vi "Periodic Tasks.vi"(8 "error in":errorcluster) -> ()   [LabVIEW 2015]
doc: "This VI runs in parallel to other tasks. It can contain as many user-defined periodic loops as you need. These can carry out PID or other sorts of timed response."
uses:
  <vilib>/Rock Robotics/WPI/Utilities/WPI_GetSetVariantRefNum.vi
  Mr. Thayer.vi
  Mr. Thayer 2.0.vi
  <vilib>/Rock Robotics/WPI/RobotDrive/WPI_RobotDriveArcadeDrive_Standard(NoSaturation).vi
  Global 3.vi
  Global 4.vi
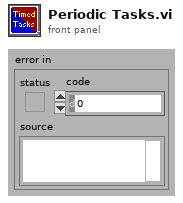
[diagram p1: front panel]
types:
  T1 = typedef "WPI_ServoDeviceRef.ctl" = cluster{"DeviceStatus":errorcluster, "PWM Channel":T2, "DeadBand":T3}
  T2 = typedef "FPGA_DIOPWMChannel.ctl" = enum8{"PWM 0", "PWM 1", "PWM 2", "PWM 3", "PWM 4", "PWM 5", "PWM 6", "PWM 7", "PWM 8", "PWM 9", "PWM MXP 0", "PWM MXP 1", "PWM MXP 2", "PWM MXP 3", "PWM MXP 4", "PWM MXP 5", "PWM MXP 6", "PWM MXP 7", "PWM MXP 8", "PWM MXP 9", "Invalid"}
  T3 = typedef "WPI_PWMDeadband.ctl" = cluster{"Name":string, "maxPositivePwm":i32, "minPositivePwm":i32, "centerPwm":i32, "maxNegativePwm":i32, "minNegativePwm":i32, "angularRange":u16}
  T4 = typedef "WPI_JoystickDevRef.ctl" = cluster{"Device":T5}
  T5 = typedef "WPI_JoystickDeviceEnum.ctl" = enum16{"USB 0", "USB 1", "USB 2", "USB 3", "USB 4", "USB 5"}
  T6 = typedef "WPI_RobotDriveDevRef.ctl" = cluster{"DevStatus":errorcluster, "Motors[]":T7[], "Square Inputs":bool, "Max Output":dbl}
  T7 = typedef "WPI_MotorControlDeviceRef.ctl" = cluster{"DeviceStatus":errorcluster, "Type":T8, "PWM":cluster{"PWM Channel":T2, "DeadBand":T3}, "CAN":cluster{"Device Number":u8, "Control Mode":T9, "Semaphore":T10, "Max Vout":dbl, "TalonSRX Control Mode":T11}, "Invert":bool}
  T8 = typedef "WPI_MotorControlType.ctl" = enum16{"PWM", "CAN", "CANTalonSRX"}
  T9 = typedef "WPI_CANJaguar_ControlMode.ctl" = enum8{"Percent VBus", "Current", "Speed", "Position", "Voltage"}
  T10 = typedef "Semaphore RefNum" = refnum<k1>
  T11 = typedef "WPI_CANTalonSRX_APIControlMode.ctl" = enum8{"Percent VBus", "Speed", "Position", "Slave", "Unchanged / Invalid", "Voltage Compensation", "Current", "Motion Profile"}
  T12 = cluster{"JoystickDevRef":T4, "RobotDriveDevRef":T6}
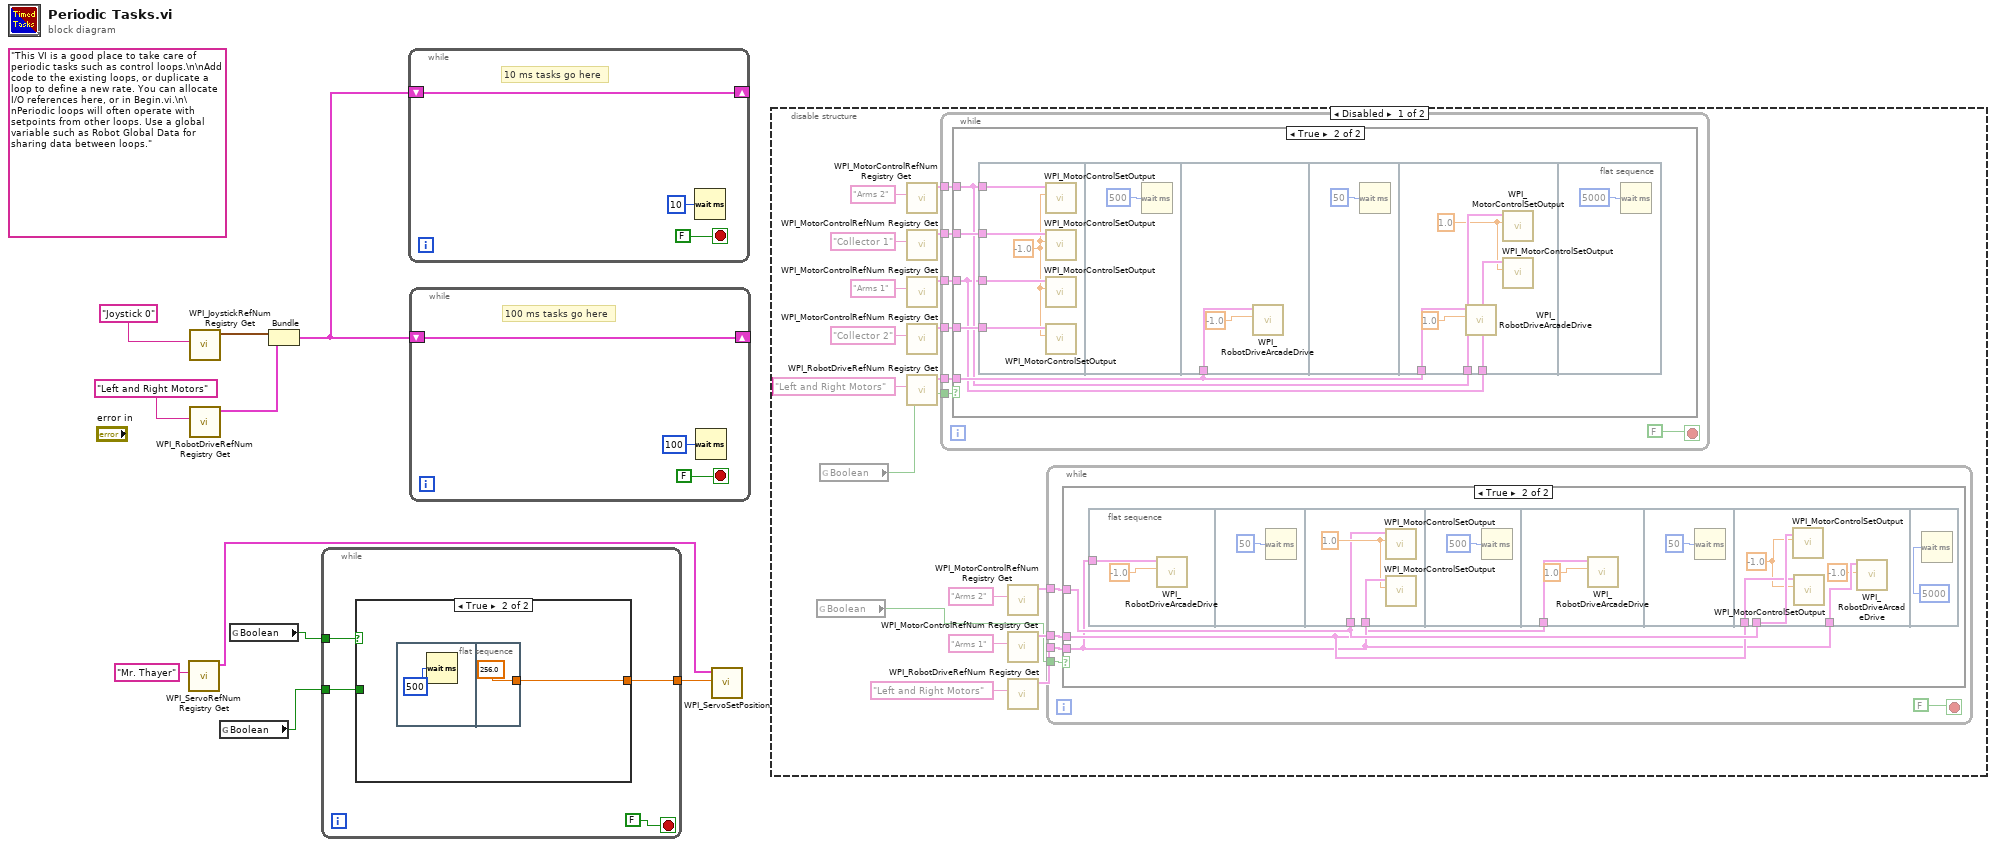
[diagram p0: block diagram]
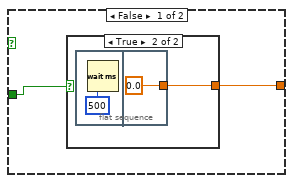
[diagram p2: hidden frame]
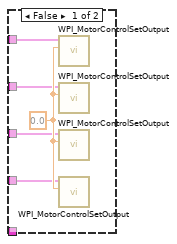
[diagram p4: hidden frame]
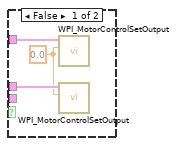
[diagram p5: hidden frame]
diagram:
  (unwired) "This VI is a good place to take care of periodic tasks such as control loops.\n\nAdd code to the existing loops, or duplicate a loop to define a new rate. You can allocate I/O references here, or in Begin.vi.\n\nPeriodic loops will often operate with setpoints from other loops. Use a global variable such as Robot Global Data for sharing data between loops."
  n1 = call <vilib>:"WPI_ServoRefNum Registry Get.vi"("refnum name"="Mr. Thayer") -> ("ServoDeviceRef"=w1:T1)  [unwired: 9 in, 1 out]
  n2 = call <vilib>:"WPI_JoystickRefNum Registry Get.vi"("refnum name"="Joystick 0") -> ("JoystickDevRef"=w8:T4)  [unwired: 1 in, 9 out]
  n3 = call <vilib>:"WPI_RobotDriveRefNum Registry Get.vi"("refnum name"="Left and Right Motors") -> ("RobotDriveDevRef"=w7:T6)  [unwired: 1 in, 9 out]
  n4 = global read "Mr. Thayer 2.0.vi" "Boolean"() -> (w3:bool)
  n5 = global read "Mr. Thayer.vi" "Boolean"() -> (w5:bool)
  n6 = Bundle("JoystickDevRef"=w8, "RobotDriveDevRef"=w7) -> (w6:T12)  [unwired: 1 out]
  n7 = while {
    tunnel: w5 -> [w14]
    tunnel: w3 -> [w13]
    tunnel: [w12] -> w2
    stop <- FALSE stop-if-true
    n8 = case shown="True" w14 {
      tunnel: w13 -> [w16 _]
      tunnel: [w15 w20] -> w12
      frame False {
        n9 = case shown="True" w16 {
          tunnel: [_ w17] -> w15
          frame False {
          }
          frame True {
            n10 = flat-sequence {
              tunnel: [0.0] -> w17
              frame #0 {
                n11 = Wait (ms)(milliseconds to wait=500) -> ()  [unwired: 1 out]
              }
              frame #1 {
              }
            }
          }
        }
      }
      frame True {
        n12 = flat-sequence {
          tunnel: [256.0] -> w20
          frame #0 {
            n13 = Wait (ms)(milliseconds to wait=500) -> ()  [unwired: 1 out]
          }
          frame #1 {
          }
        }
      }
    }
  }
  n14 = while {
    shift-right: [w23] -> _
    shift-left: w6 -> [w23]
    stop <- FALSE stop-if-true
    # "10 ms tasks go here"
    n15 = Wait (ms)(milliseconds to wait=u32 10) -> ()  [unwired: 1 out]
  }
  n16 = while {
    shift-right: [w26] -> _
    shift-left: w6 -> [w26]
    stop <- FALSE stop-if-true
    # "100 ms tasks go here"
    n17 = Wait (ms)(milliseconds to wait=u32 100) -> ()  [unwired: 1 out]
  }
  n18 = call <vilib>:"WPI_ServoSetPosition.vi"("Position"=w2, "ServoDeviceRef"=w1) -> ()  [unwired: 8 in, 2 out]
  n19 = disable-structure shown="Disabled" {
    frame Disabled {
      n20 = global read "Global 4.vi" "Boolean"() -> (w29:bool)
      n21 = global read "Global 3.vi" "Boolean"() -> (w36:bool)
      n22 = call <vilib>:"WPI_MotorControlRefNum Registry Get.vi"("refnum name"="Arms 2") -> ("MotorControlDevRef"=w43:T7)  [unwired: 9 in, 1 out]
      n23 = call <vilib>:"WPI_MotorControlRefNum Registry Get.vi"("refnum name"="Collector 1") -> ("MotorControlDevRef"=w46:T7)  [unwired: 9 in, 1 out]
      n24 = call <vilib>:"WPI_MotorControlRefNum Registry Get.vi"("refnum name"="Arms 1") -> ("MotorControlDevRef"=w44:T7)  [unwired: 9 in, 1 out]
      n25 = call <vilib>:"WPI_MotorControlRefNum Registry Get.vi"("refnum name"="Collector 2") -> ("MotorControlDevRef"=w45:T7)  [unwired: 9 in, 1 out]
      n26 = call <vilib>:"WPI_RobotDriveRefNum Registry Get.vi"("refnum name"="Left and Right Motors") -> ("RobotDriveDevRef"=w37:T6)  [unwired: 9 in, 1 out]
      n27 = while {
        tunnel: w46 -> [w53]
        tunnel: w45 -> [w52]
        tunnel: w44 -> [w51]
        tunnel: w43 -> [w50]
        tunnel: w37 -> [w49]
        tunnel: w36 -> [w48]
        stop <- FALSE stop-if-true
        n28 = case shown="True" w48 {
          tunnel: w53 -> [w57 w63]
          tunnel: w52 -> [w56 w62]
          tunnel: w51 -> [w55 w59]
          tunnel: w50 -> [w54 w60]
          tunnel: w49 -> [_ w61]
          frame False {
            w58 = 0.0
            n29 = call <vilib>:"WPI_MotorControlSetOutput.vi"("Output"=w58, "MotorControlDevRef"=w54) -> ()  [unwired: 7 in, 3 out]
            n30 = call <vilib>:"WPI_MotorControlSetOutput.vi"("Output"=w58, "MotorControlDevRef"=w57) -> ()  [unwired: 7 in, 3 out]
            n31 = call <vilib>:"WPI_MotorControlSetOutput.vi"("Output"=w58, "MotorControlDevRef"=w55) -> ()  [unwired: 7 in, 3 out]
            n32 = call <vilib>:"WPI_MotorControlSetOutput.vi"("Output"=w58, "MotorControlDevRef"=w56) -> ()  [unwired: 7 in, 3 out]
          }
          frame True {
            n33 = flat-sequence {
              tunnel: w63 -> [w68]
              tunnel: w62 -> [w67]
              tunnel: w59 -> [w66]
              tunnel: w60 -> [w65]
              tunnel: w61 -> [w71]
              tunnel: w61 -> [w77]
              tunnel: w60 -> [w75]
              tunnel: w59 -> [w74]
              frame #0 {
                w64 = -1.0
                n34 = call <vilib>:"WPI_MotorControlSetOutput.vi"("Output"=w64, "MotorControlDevRef"=w65) -> ()  [unwired: 7 in, 3 out]
                n35 = call <vilib>:"WPI_MotorControlSetOutput.vi"("Output"=w64, "MotorControlDevRef"=w68) -> ()  [unwired: 7 in, 3 out]
                n36 = call <vilib>:"WPI_MotorControlSetOutput.vi"("Output"=w64, "MotorControlDevRef"=w66) -> ()  [unwired: 7 in, 3 out]
                n37 = call <vilib>:"WPI_MotorControlSetOutput.vi"("Output"=w64, "MotorControlDevRef"=w67) -> ()  [unwired: 7 in, 3 out]
              }
              frame #1 {
                n38 = Wait (ms)(milliseconds to wait=500) -> ()  [unwired: 1 out]
              }
              frame #2 {
                n39 = call-poly <vilib>:"WPI_RobotDriveArcadeDrive.vi"("X axis value"=-1.0, "RobotDriveDevRef"=w71) -> ()  [unwired: 7 in, 3 out]
              }
              frame #3 {
                n40 = Wait (ms)(milliseconds to wait=50) -> ()  [unwired: 1 out]
              }
              frame #4 {
                w73 = 1.0
                n41 = call-poly <vilib>:"WPI_RobotDriveArcadeDrive.vi"("X axis value"=1.0, "RobotDriveDevRef"=w77) -> ()  [unwired: 7 in, 3 out]
                n42 = call <vilib>:"WPI_MotorControlSetOutput.vi"("Output"=w73, "MotorControlDevRef"=w75) -> ()  [unwired: 7 in, 3 out]
                n43 = call <vilib>:"WPI_MotorControlSetOutput.vi"("Output"=w73, "MotorControlDevRef"=w74) -> ()  [unwired: 7 in, 3 out]
              }
              frame #5 {
                n44 = Wait (ms)(milliseconds to wait=5000) -> ()  [unwired: 1 out]
              }
            }
          }
        }
      }
      n45 = call <vilib>:"WPI_MotorControlRefNum Registry Get.vi"("refnum name"="Arms 2") -> ("MotorControlDevRef"=w31:T7)  [unwired: 9 in, 1 out]
      n46 = call <vilib>:"WPI_MotorControlRefNum Registry Get.vi"("refnum name"="Arms 1") -> ("MotorControlDevRef"=w35:T7)  [unwired: 9 in, 1 out]
      n47 = call <vilib>:"WPI_RobotDriveRefNum Registry Get.vi"("refnum name"="Left and Right Motors") -> ("RobotDriveDevRef"=w32:T6)  [unwired: 9 in, 1 out]
      n48 = while {
        tunnel: w35 -> [w83]
        tunnel: w32 -> [w82]
        tunnel: w31 -> [w81]
        tunnel: w29 -> [w80]
        stop <- FALSE stop-if-true
        n49 = case shown="True" w80 {
          tunnel: w83 -> [w86 w88]
          tunnel: w82 -> [_ w87]
          tunnel: w81 -> [w85 w89]
          frame False {
            w84 = 0.0
            n50 = call <vilib>:"WPI_MotorControlSetOutput.vi"("Output"=w84, "MotorControlDevRef"=w85) -> ()  [unwired: 7 in, 3 out]
            n51 = call <vilib>:"WPI_MotorControlSetOutput.vi"("Output"=w84, "MotorControlDevRef"=w86) -> ()  [unwired: 7 in, 3 out]
          }
          frame True {
            n52 = flat-sequence {
              tunnel: w87 -> [w91]
              tunnel: w88 -> [w95]
              tunnel: w89 -> [w93]
              tunnel: w87 -> [w98]
              tunnel: w89 -> [w104]
              tunnel: w88 -> [w103]
              tunnel: w87 -> [w101]
              frame #0 {
                n53 = call-poly <vilib>:"WPI_RobotDriveArcadeDrive.vi"("X axis value"=-1.0, "RobotDriveDevRef"=w91) -> ()  [unwired: 7 in, 3 out]
              }
              frame #1 {
                n54 = Wait (ms)(milliseconds to wait=50) -> ()  [unwired: 1 out]
              }
              frame #2 {
                w94 = 1.0
                n55 = call <vilib>:"WPI_MotorControlSetOutput.vi"("Output"=w94, "MotorControlDevRef"=w93) -> ()  [unwired: 7 in, 3 out]
                n56 = call <vilib>:"WPI_MotorControlSetOutput.vi"("Output"=w94, "MotorControlDevRef"=w95) -> ()  [unwired: 7 in, 3 out]
              }
              frame #3 {
                n57 = Wait (ms)(milliseconds to wait=500) -> ()  [unwired: 1 out]
              }
              frame #4 {
                n58 = call-poly <vilib>:"WPI_RobotDriveArcadeDrive.vi"("X axis value"=1.0, "RobotDriveDevRef"=w98) -> ()  [unwired: 7 in, 3 out]
              }
              frame #5 {
                n59 = Wait (ms)(milliseconds to wait=50) -> ()  [unwired: 1 out]
              }
              frame #6 {
                w102 = -1.0
                n60 = call <vilib>:"WPI_MotorControlSetOutput.vi"("Output"=w102, "MotorControlDevRef"=w104) -> ()  [unwired: 7 in, 3 out]
                n61 = call <vilib>:"WPI_MotorControlSetOutput.vi"("Output"=w102, "MotorControlDevRef"=w103) -> ()  [unwired: 7 in, 3 out]
                n62 = call-poly <vilib>:"WPI_RobotDriveArcadeDrive.vi"("X axis value"=-1.0, "RobotDriveDevRef"=w101) -> ()  [unwired: 7 in, 3 out]
              }
              frame #7 {
                n63 = Wait (ms)(milliseconds to wait=5000) -> ()  [unwired: 1 out]
              }
            }
          }
        }
      }
    }
    frame Enabled {
    }
  }
